vi "Simple Reader.vi"(8 "error in (no error)":errorcluster, 11 "LR-700 Driver in":refnum<class "LR-700 Driver.lvclass">) -> (0 "error out":errorcluster, 2 "Signals":dbl[](array[numeric]), 3 "LR-700 Driver out":refnum<class "LR-700 Driver.lvclass">)   [LabVIEW 2019, in "LR-700 Driver.lvclass"]
uses:
  LR-700 Driver.lvclass
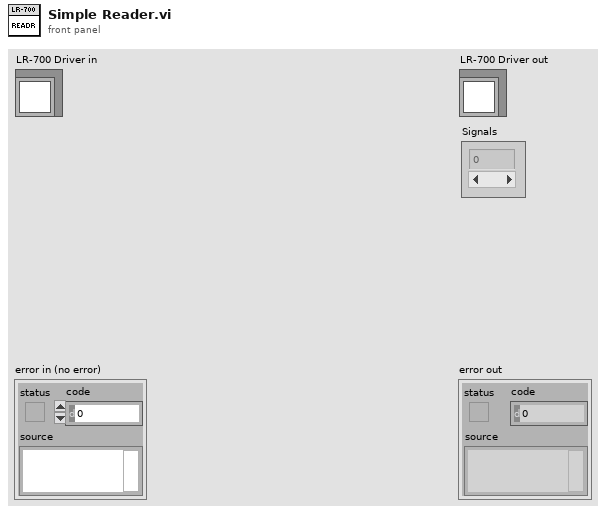
[diagram p1: front panel]
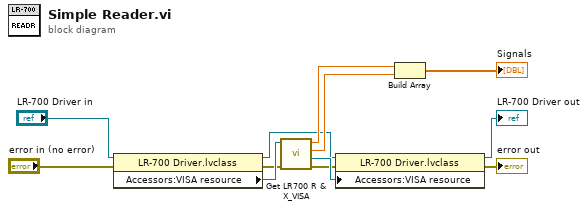
[diagram p0: block diagram]
diagram:
  n1 = property class="LR-700 Driver.lvclass"(reference="LR-700 Driver in", error in="error in (no error)") -> (reference out=w3:refnum<class "LR-700 Driver.lvclass">, error out=w2:errorcluster, "Accessors:VISA resource"=w8:refnum<visa-resource-name>)
  n2 = call "Get LR700 R & X_VISA.vi"("error in (no error)"=w2, "VISA resource name"=w8) -> ("error out"=w1:errorcluster, "VISA resource name out"=w7:refnum<visa-resource-name>, "X"=w5:dbl, "Resistance"=w6:dbl)  [unwired: 2 in]
  n3 = property class="LR-700 Driver.lvclass"(reference=w3, error in=w1, "Accessors:VISA resource"=w7) -> (reference out=→"LR-700 Driver out":refnum<class "LR-700 Driver.lvclass">, error out=→"error out":errorcluster)
  n4 = Build Array(w6, w5) -> (→"Signals":dbl[])
